vi "determine test case.vi"(6 "error in":errorcluster, 7 "file path (dialog if empty)":path, 10 "Test this case?":bool, 11 "Test Matrix":i32(listbox)) -> (0 "error out":errorcluster, 1 "Test Matrix Data":T2, 3 "Test Case Cluster":T1)   [LabVIEW 2013]
uses:
  Controls/data.ctl
  Controls/Test Case.ctl
  <vilib>/Utility/miscctls.llb/LVRowAndColumnTypeDef.ctl
  <vilib>/Utility/file.llb/Read From Spreadsheet File (string).vi
panel:
  # "Choose a test case from the test matrix"
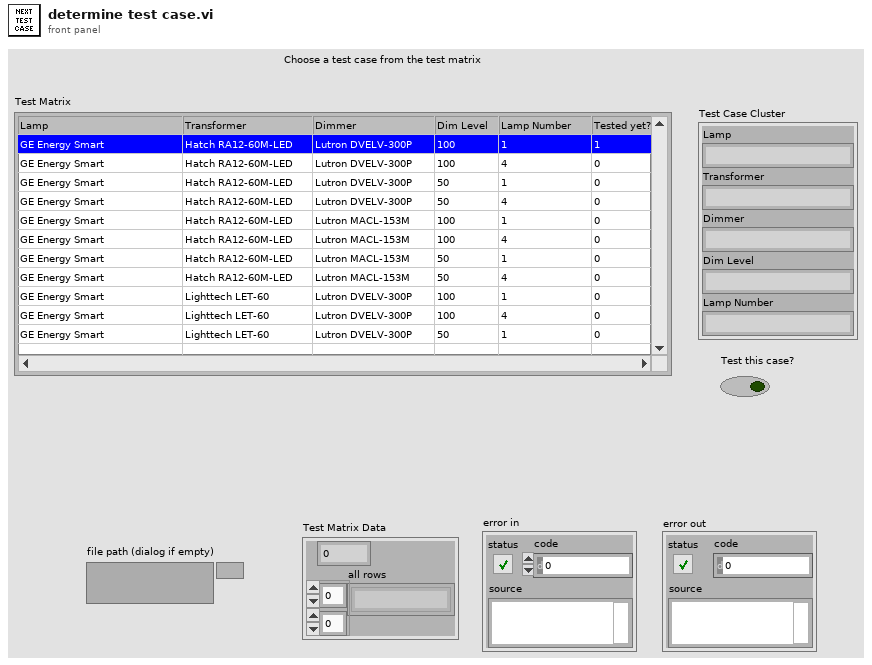
[diagram p1: front panel]
types:
  T1 = typedef "Test Case.ctl" = cluster{"Lamp":string, "Transformer":string, "Dimmer":string, "Dim Level":string, "Lamp Number":string}
  T2 = typedef "data.ctl" = cluster{"index":i32, "all rows":string[][]}
  T3 = typedef "LVRowAndColumnTypeDef.ctl" = cluster{"Row":i32, "Column":i32}
  T4 = cluster{"Test Matrix":i32, "all rows":string[][]}
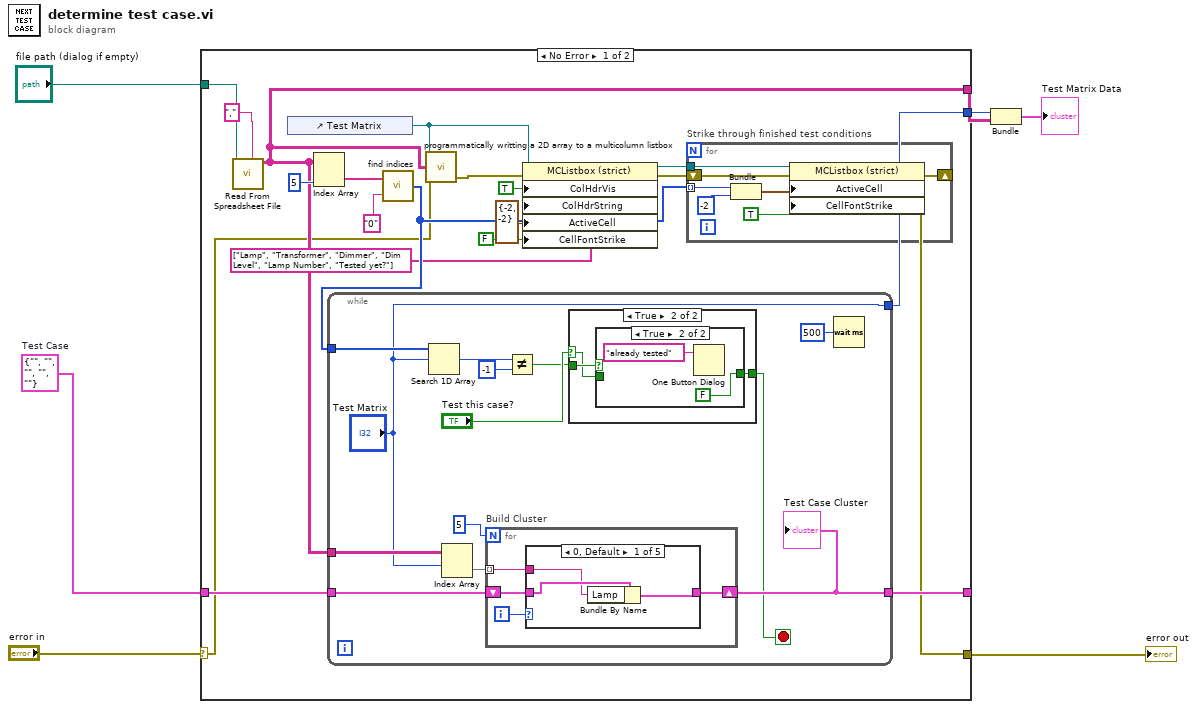
[diagram p0: block diagram]
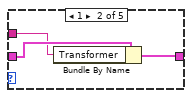
[diagram p4: hidden frame]
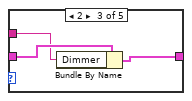
[diagram p5: hidden frame]
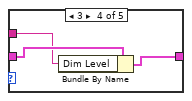
[diagram p6: hidden frame]
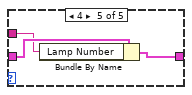
[diagram p7: hidden frame]
diagram:
  w1 = T1 {"Lamp"="", "Transformer"="", "Dimmer"="", "Dim Level"="", "Lamp Number"=""}  # Test Case
  n1 = case shown="No Error" "error in" {
    selector: "error in" -> [w17 w74]
    tunnel: [w25 _] -> w4
    tunnel: [w20 _] -> w3
    tunnel: "file path (dialog if empty)" -> [w24 _]
    tunnel: [w16 w74] -> w5
    tunnel: w1 -> [w23 _]
    tunnel: [w22 _] -> _
    frame No Error {
      n2 = call-poly <vilib>:"Read From Spreadsheet File.vi"("delimiter (\\t)"="," ("delimiter (\\t)"), "file path (dialog if empty)"=w24) -> ("all rows"=w20:string[][])  [unwired: 5 in, 4 out]
      n3 = control-ref of="Test Matrix"() -> (w13:refnum<vi>)
      n4 = Index Array(array=w20, index (col)=5 ("disabled index (col)")) -> (element=w21:string[])  [unwired: 1 in]
      n5 = call "find indices.vi"("value to compare"="0", "search array"=w21) -> ("indices"=w18:i32[])
      n6 = while {
        tunnel: w23 -> [w38]
        tunnel: [w36] -> w22
        tunnel: ["Test Matrix"] -> w25
        tunnel: w20 -> [w37]
        tunnel: w18 -> [w35]
        stop <- w31 stop-if-true
        n7 = Search 1D Array(1D array=w35, element="Test Matrix") -> (index of element=w33:i32)  [unwired: 1 in]
        n8 = Index Array(array=w37, index (row)="Test Matrix") -> (element=w40:string[])  [unwired: 1 in]
        n9 = for "Build Cluster" {
          N: 5 -> [_]
          tunnel: w40 -> [w51] mode=indexing
          shift-right: [w48] -> w36
          shift-left: w38 -> [w49]
          i -> [w50]
          n10 = case shown="0, Default" w50 {
            tunnel: w51 -> [w52 w55 w58 w61 w64]
            tunnel: w49 -> [w54 w56 w60 w63 w66]
            tunnel: [w53 w57 w59 w62 w65] -> w48
            frame 0, Default {
              n11 = Bundle By Name(cluster=w54, "Lamp"=w52) -> (w53:T1)
            }
            frame 1 {
              n12 = Bundle By Name(cluster=w56, "Transformer"=w55) -> (w57:T1)
            }
            frame 2 {
              n13 = Bundle By Name(cluster=w60, "Dimmer"=w58) -> (w59:T1)
            }
            frame 3 {
              n14 = Bundle By Name(cluster=w63, "Dim Level"=w61) -> (w62:T1)
            }
            frame 4 {
              n15 = Bundle By Name(cluster=w66, "Lamp Number"=w64) -> (w65:T1)
            }
          }
        }
        "Test Case Cluster" <- w36
        n16 = Not Equal?(x=w33, y=-1) -> (x != y?=w28:bool)
        n17 = case shown="True" "Test this case?" {
          selector: "Test this case?" -> [w41 w42]
          tunnel: [w41 w44] -> w31
          tunnel: w28 -> [_ w43]
          frame False {
          }
          frame True {
            n18 = case shown="True" w43 {
              tunnel: [w45 FALSE] -> w44
              tunnel: w42 -> [w45 _]
              frame False {
              }
              frame True {
                n19 = One Button Dialog(message="already tested") -> ()  [unwired: 1 in, 1 out]
              }
            }
          }
        }
        n20 = Wait (ms)(milliseconds to wait=u32 500) -> ()  [unwired: 1 out]
      }
      n21 = call "programmatically writting a 2D array to a multicolumn listbox.vi"("MCListbox Refnum"=w13, "Input 2D Array"=w20, "error in"=w17) -> ("error out"=w15:errorcluster)  [unwired: 4 in, 2 out]
      n22 = property class="MCListbox (strict)"(reference=w13, error in=w15, "ColHdrVis"=TRUE ("Visible Items:Column Headers Visible"), "ColHdrString"=string[] ["Lamp", "Transformer", "Dimmer", "Dim Level", "Lamp Number", "Tested yet?"] ("Column Header Strings[]"), "ActiveCell"=T3 {"Row"=-2, "Column"=-2} ("Active Cell:Active Cell"), "CellFontStrike"=FALSE ("Active Cell:Cell Font:Strikeout")) -> (reference out=w12:refnum<vi>, error out=w14:errorcluster)
      n23 = for "Strike through finished test conditions" {
        tunnel: w12 -> [w73]
        tunnel: w18 -> [w70] mode=indexing
        shift-right: [w68] -> w16
        shift-left: w14 -> [w67]
        n24 = Bundle(w70, -2) -> (w69:cluster{i32, i32})  [unwired: 1 in]
        n25 = property class="MCListbox (strict)"(reference=w73, error in=w67, "ActiveCell"=w69, "CellFontStrike"=TRUE ("Active Cell:Cell Font:Strikeout")) -> (error out=w68:errorcluster)  [unwired: 1 out]
      }
    }
    frame Error {
    }
  }
  "error out" <- w5
  n26 = Bundle("Test Matrix"=w4, "all rows"=w3) -> (→"Test Matrix Data":T4)  [unwired: 1 in]
